vi "22_Operation using case structure.vi"() -> ()   [LabVIEW 2022 SP3]
panel:
  out "Result":dbl
  in  "Operation":dbl
  in  "B":dbl
  in  "A":dbl
  # "Develop a HMI to perform operation using case structure\nif (1): Addition\nif (2) Subtraction\nif (3): Multiplication\nif (4): Division"
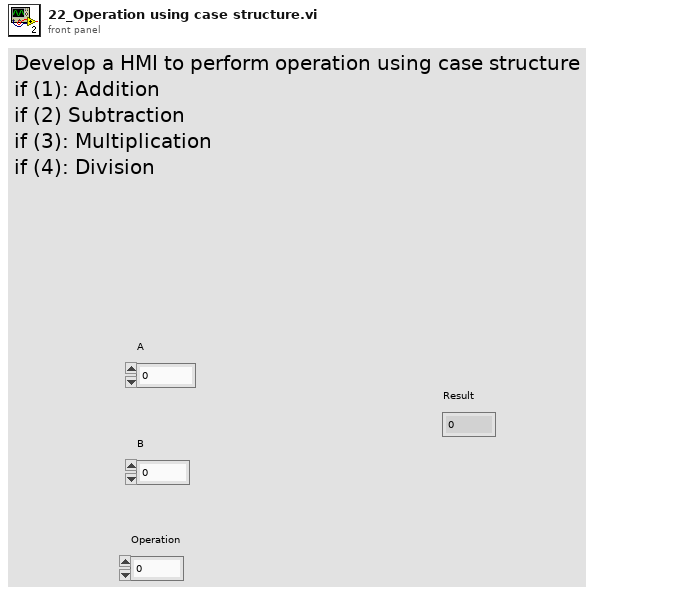
[diagram p1: front panel]
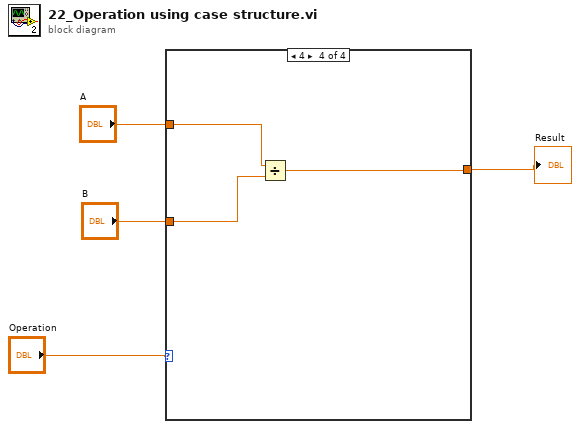
[diagram p0: block diagram]
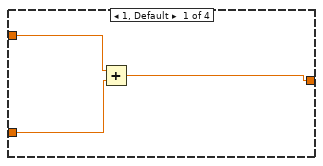
[diagram p2: hidden frame]
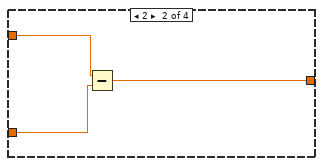
[diagram p3: hidden frame]
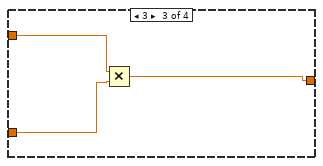
[diagram p4: hidden frame]
diagram:
  n1 = case shown="4" "Operation" {
    tunnel: "A" -> [w7 w10 w13 w16]
    tunnel: "B" -> [w6 w9 w12 w15]
    tunnel: [w5 w8 w11 w14] -> w1
    frame 1, Default {
      n2 = Add(x=w7, y=w6) -> (x+y=w5:dbl)
    }
    frame 2 {
      n3 = Subtract(x=w10, y=w9) -> (x-y=w8:dbl)
    }
    frame 3 {
      n4 = Multiply(x=w13, y=w12) -> (x*y=w11:dbl)
    }
    frame 4 {
      n5 = Divide(x=w16, y=w15) -> (x/y=w14:dbl)
    }
  }
  "Result" <- w1
